vi "SMO.TopLevel.TestLauncher.vi"() -> ()   [LabVIEW 2013]
uses:
  src/SMO/Typedefs/SMOState --Enum.ctl
  SMO.TopLevel.lvclass
  src/SMO/SMO.lvclass
  src/Registry/Registry-SMO.lvclass
panel:
  in  "Registered SMOs":i32(listbox)
  in  "Check Context":bool
  out "A Name":string
  in  "Start Nested":bool
  in  "Stop":bool
  # "SMO Test Launcher"
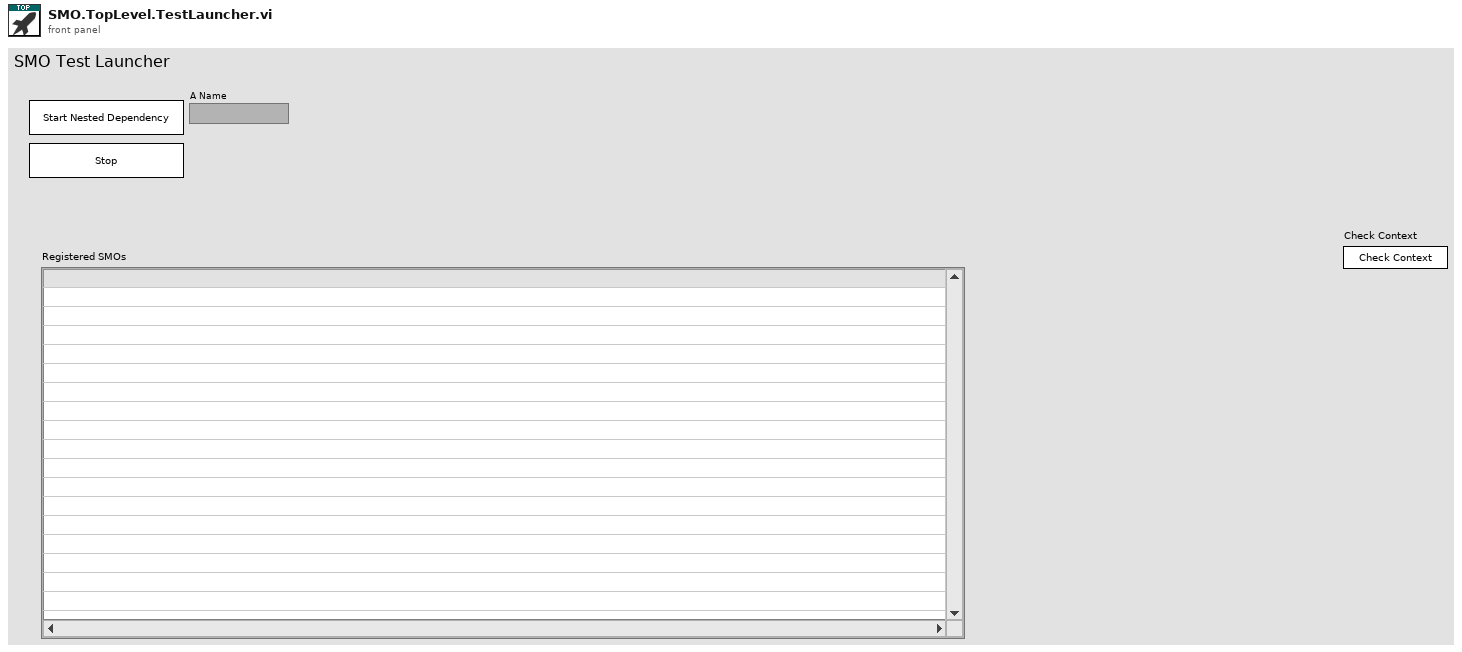
[diagram p1: front panel]
types:
  T1 = typedef "SMO.lvclass/SMOState --Enum.ctl" = enum16{"unknown", "Created", "Started", "Stopped"}
  T2 = enum32{"invalid app kind", "Development System", "Run Time System", "Student Edition", "Embedded LabVIEW", "Evaluation", "Custom"}
  T3 = enum32{"Invalid", "Standard", "Closed", "Hidden", "Minimized", "Maximized"}
  T4 = cluster{"Core":cluster{"Current VI Reference":refnum<vi>, "Close Panel on Exit?":bool}, "SMO":refnum<class "SMO.TopLevel.lvclass">, "Your string data":string}
  T5 = cluster{"Current VI Reference":refnum<vi>, "Close Panel on Exit?":bool}
  T6 = typedef "Registry-SMO.lvclass/PublicRegistryEvents--Cluster.ctl" = cluster{"Register Event":refnum<user-event>, "Unregister Event":refnum<user-event>}
  T7 = typedef "SMO.lvclass/Public Events.ctl" = cluster{"Error":refnum<user-event>, "State":refnum<user-event>}
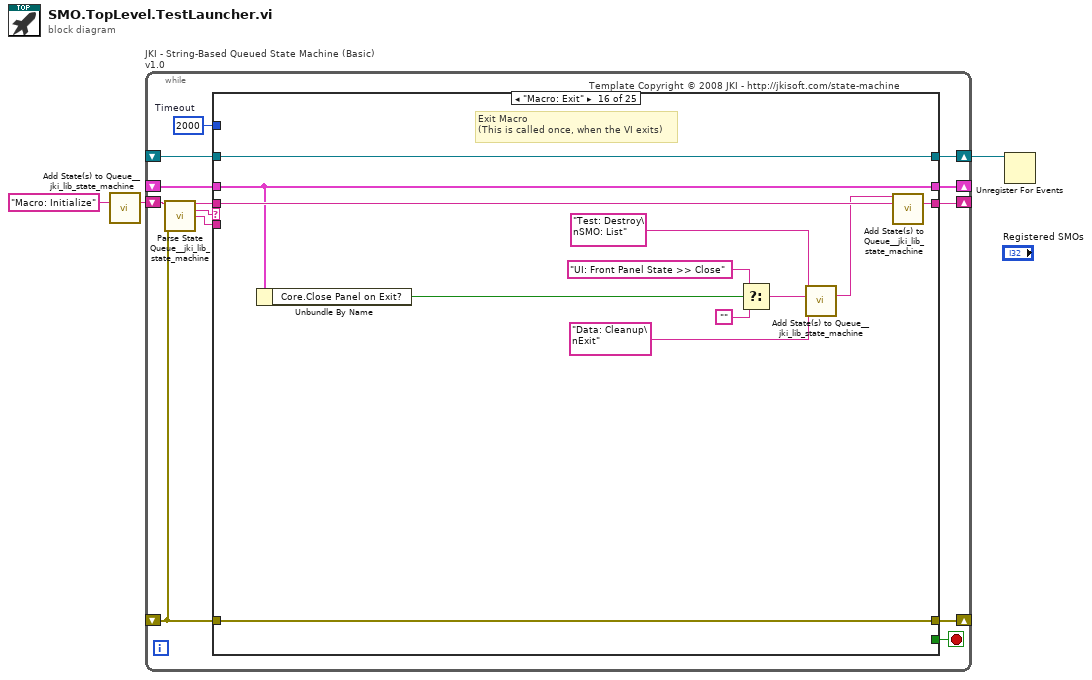
[diagram p0: block diagram]
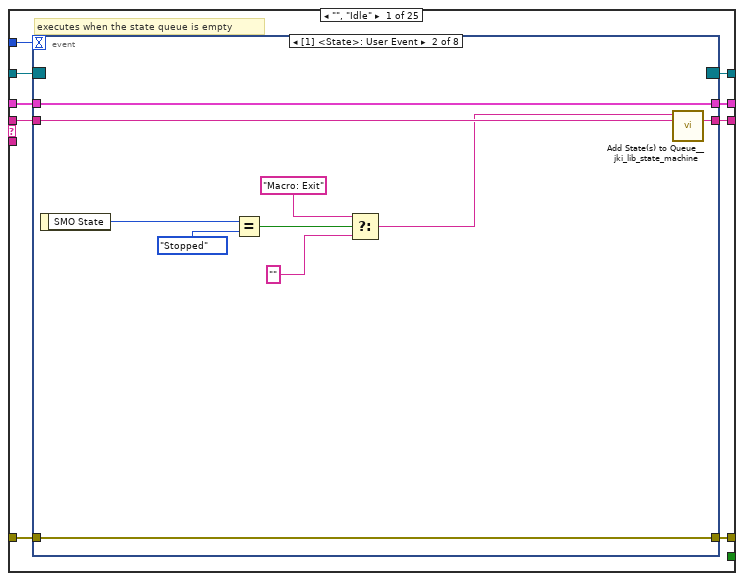
[diagram p2: hidden frame]
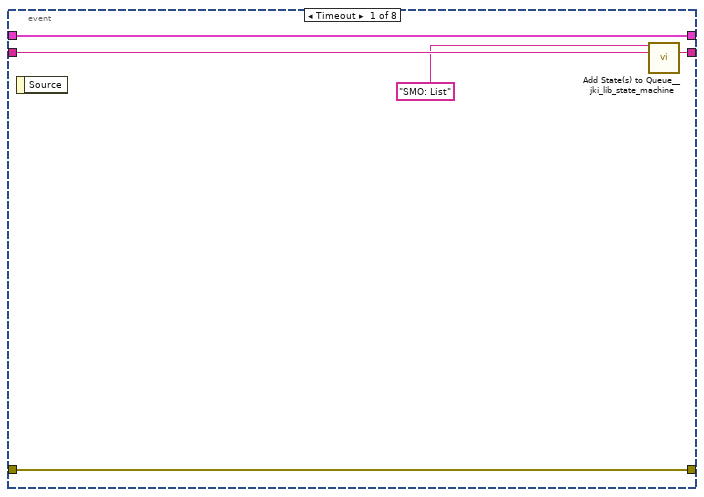
[diagram p3: hidden frame]
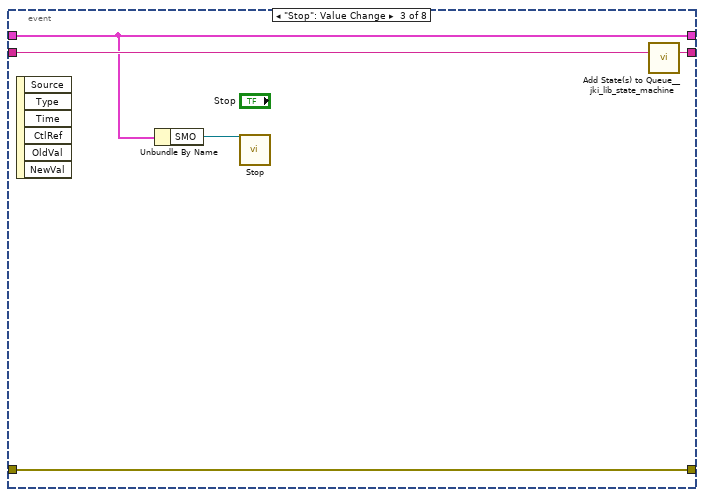
[diagram p4: hidden frame]
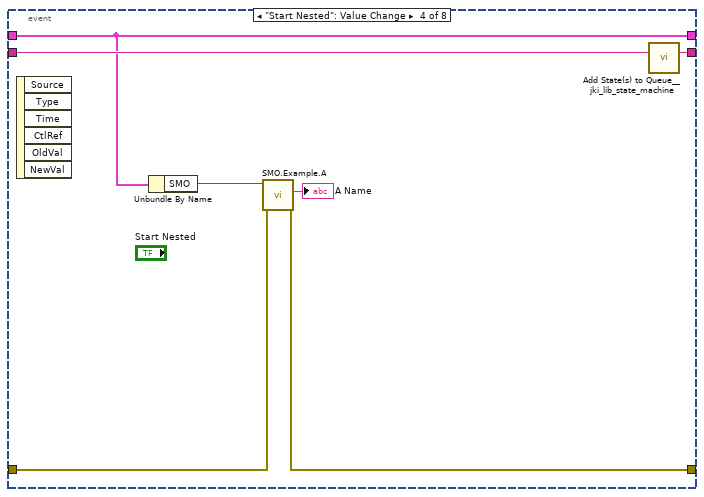
[diagram p5: hidden frame]
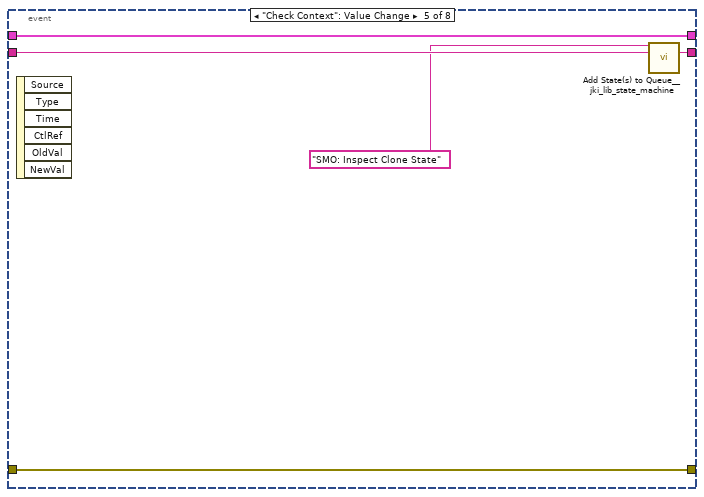
[diagram p6: hidden frame]
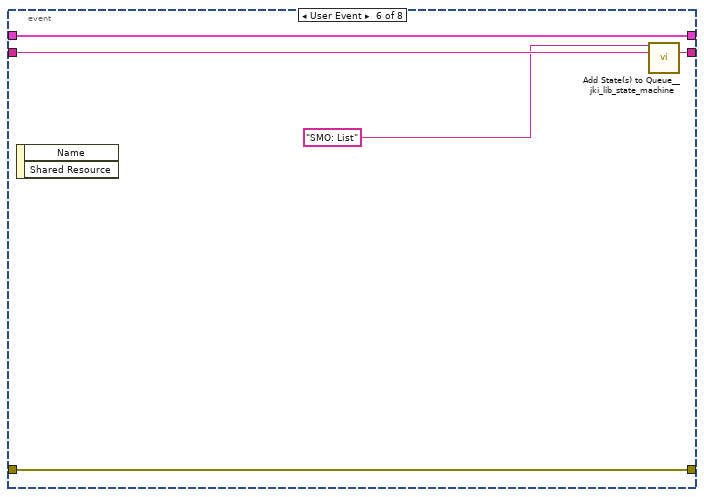
[diagram p7: hidden frame]
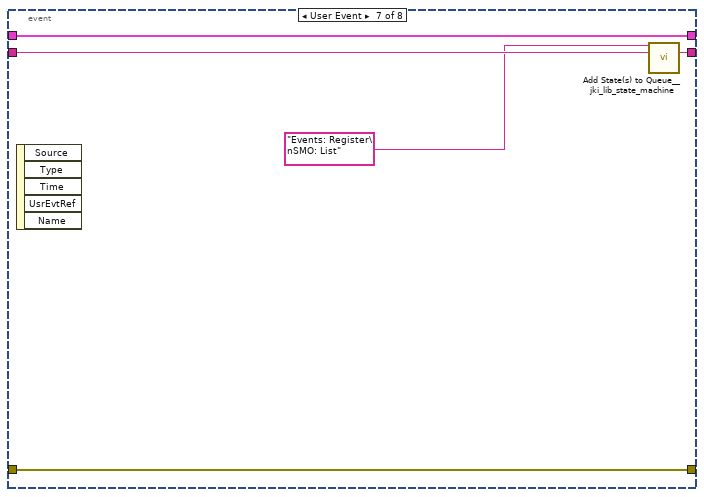
[diagram p8: hidden frame]
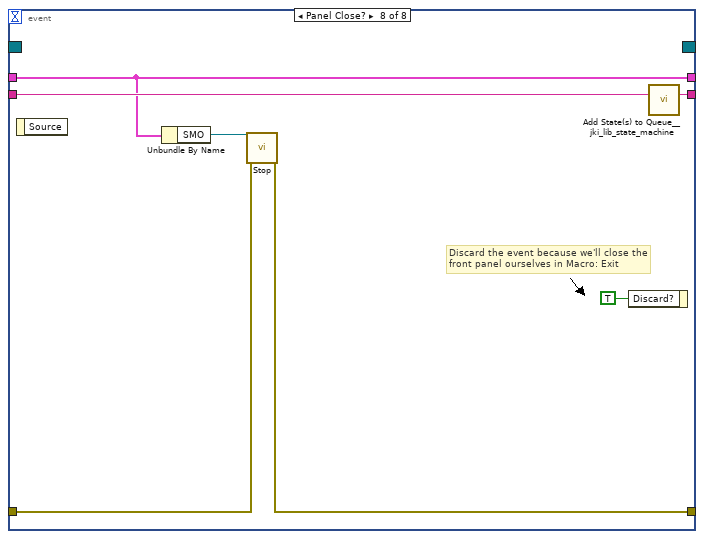
[diagram p9: hidden frame]
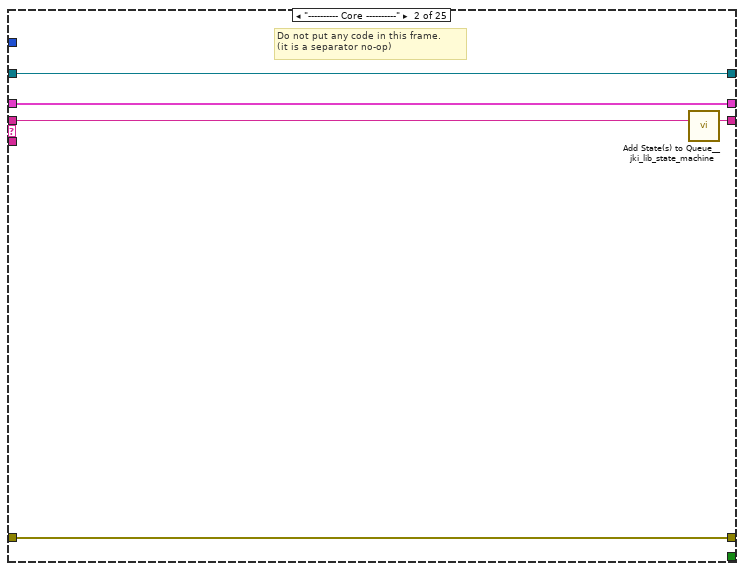
[diagram p10: hidden frame]
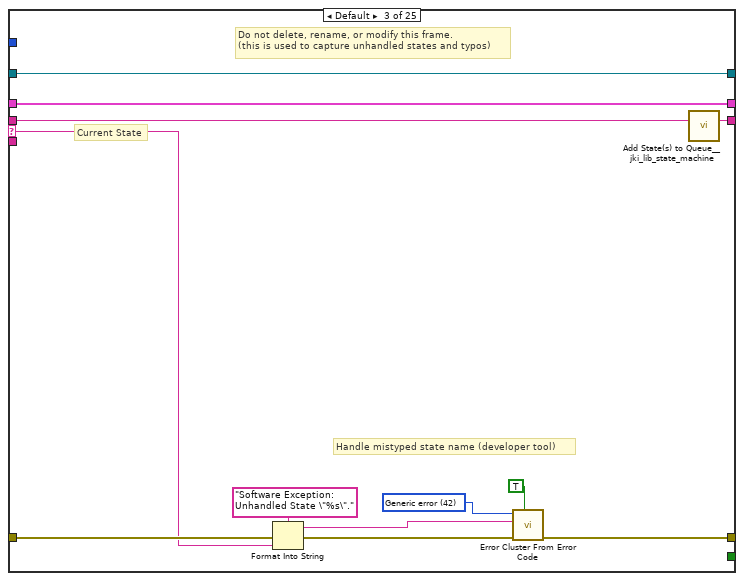
[diagram p11: hidden frame]
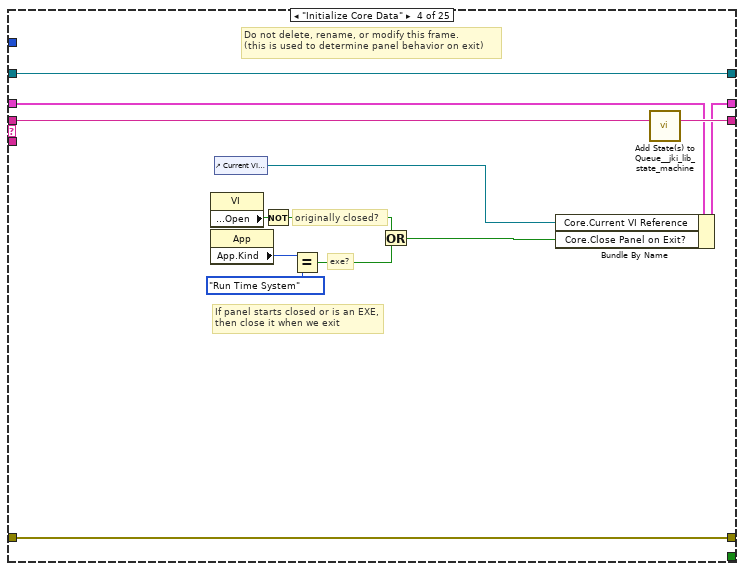
[diagram p12: hidden frame]
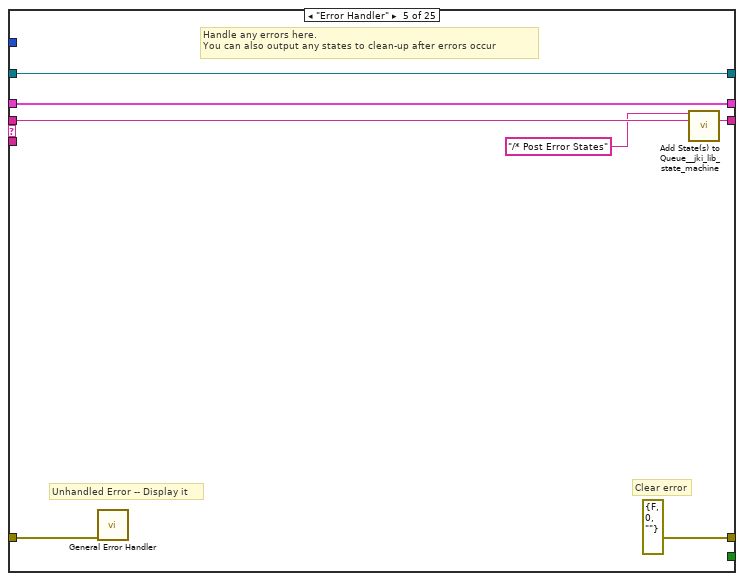
[diagram p13: hidden frame]
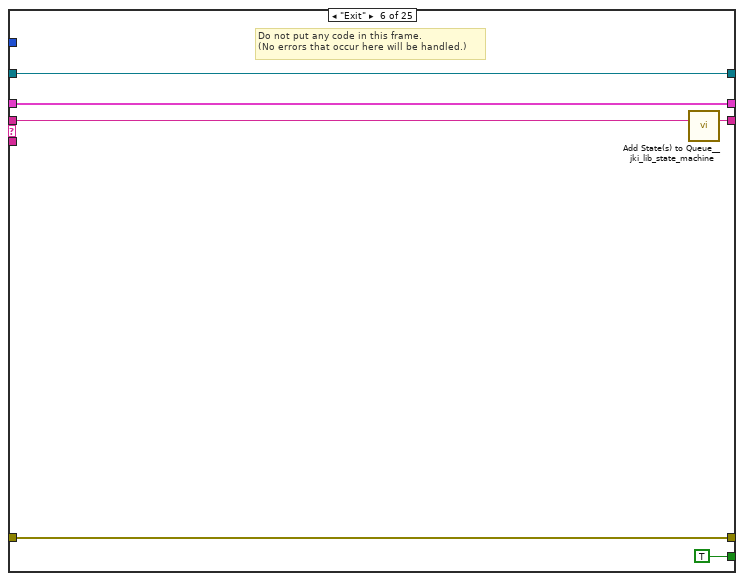
[diagram p14: hidden frame]
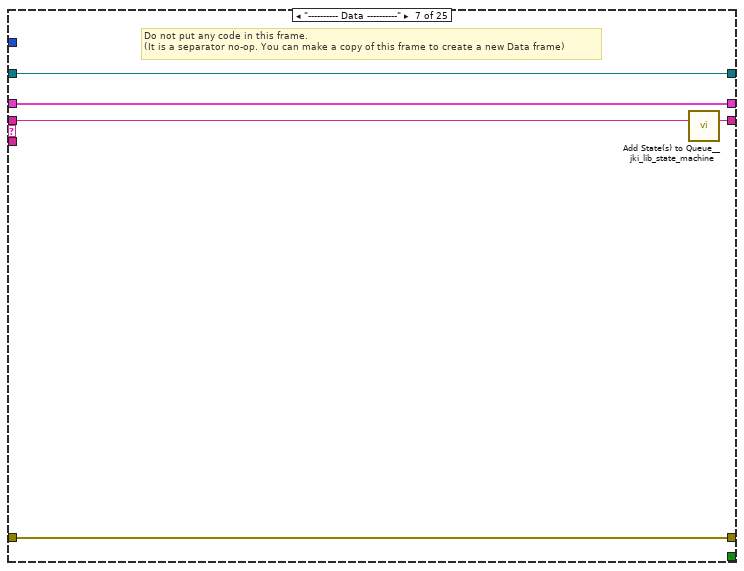
[diagram p15: hidden frame]
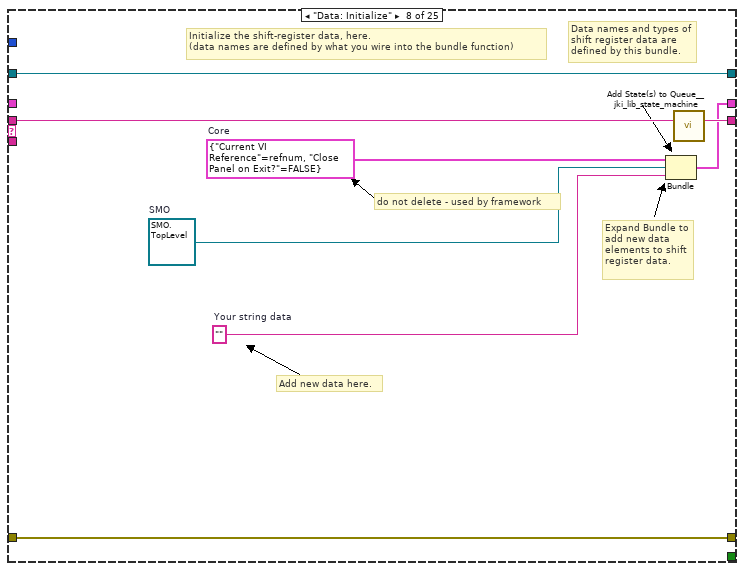
[diagram p16: hidden frame]
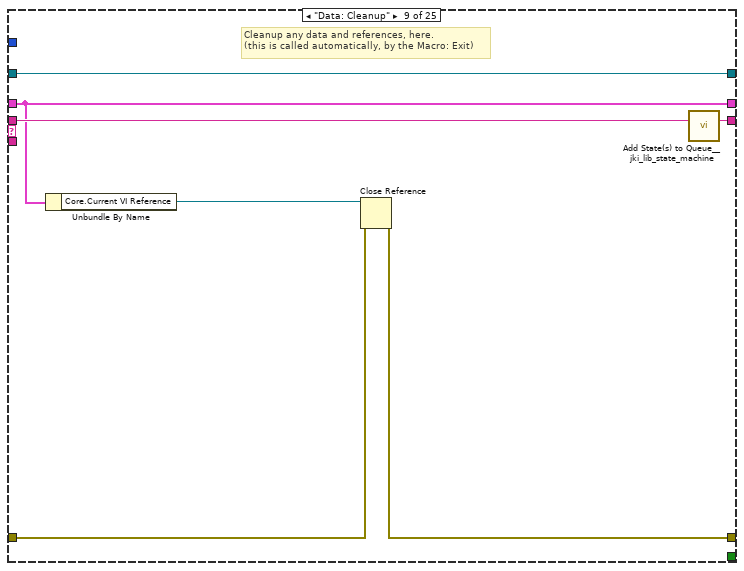
[diagram p17: hidden frame]
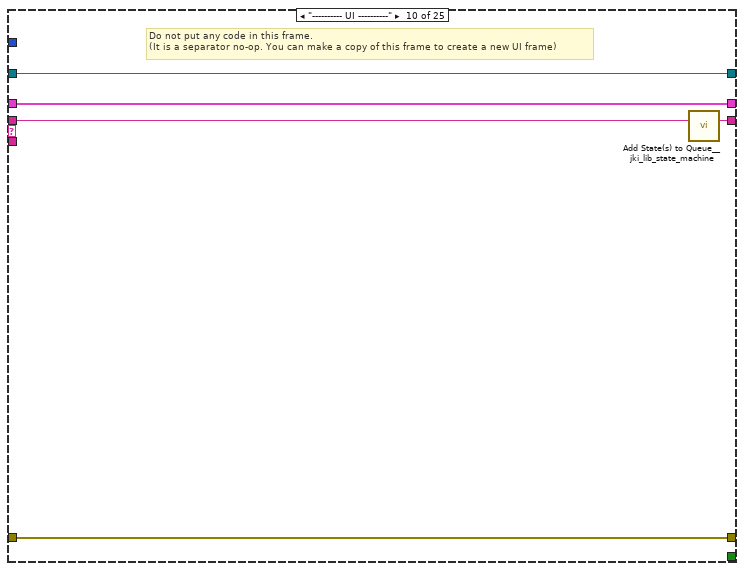
[diagram p18: hidden frame]
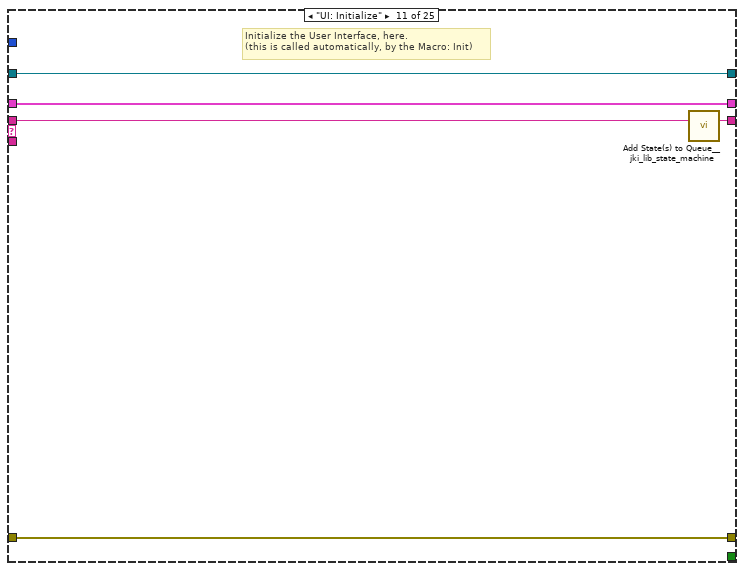
[diagram p19: hidden frame]
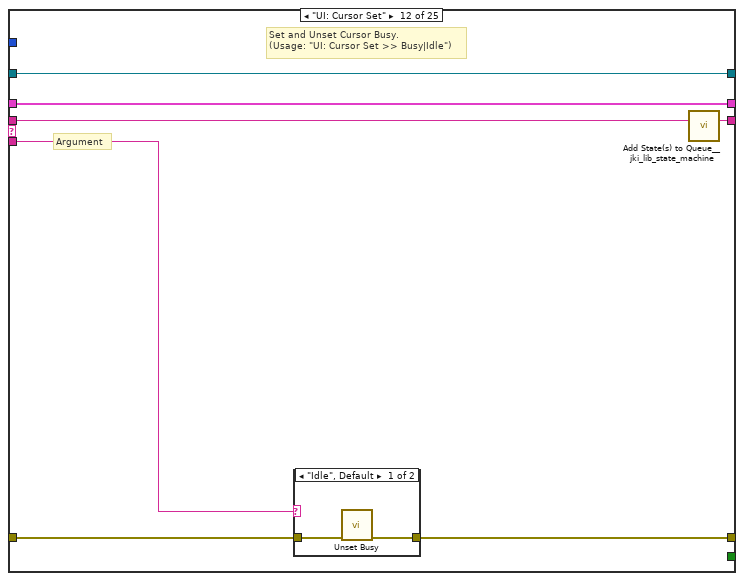
[diagram p20: hidden frame]
diagram:
  n1 = call <vilib>:"Add State(s) to Queue__jki_lib_state_machine.vi"("State(s) in (\"\")"="Macro: Initialize") -> ("States Out"=w1:string)  [unwired: 14 in]
  n2 = while "JKI - String-Based Queued State Machine (Basic) v1.0" {
    shift-right: [w9] -> _
    shift-left: _ -> [w8]
    shift-right: [w12] -> _
    shift-left: _ -> [w6]
    shift-right: [w11] -> _
    shift-left: w1 -> [w13]
    shift-right: [w4] -> w3
    shift-left: _ -> [w5]
    stop <- w10 stop-if-true
    w7 = 2000  # Timeout
    # "Template Copyright © 2008 JKI - http://jkisoft.com/state-machine"
    n3 = call <vilib>:"Parse State Queue__jki_lib_state_machine.vi"("State Queue"=w13, "Error In (no error)"=w6) -> ("Remaining States"=w15:string, "Current State"=w16:string, "Arguments"=w14:string)  [unwired: 11 in]
    n4 = case shown="\"Macro: Exit\"" w16 {
      selector: w16 -> [_ _ w81 _ _ _ _ _ _ _ _ _ _ _ _ _ _ _ _ _ _ _ _ _ _]
      tunnel: w15 -> [w25 w79 w85 w104 w111 w117 w122 w130 w137 w142 w147 w154 w166 w193 w199 w211 w216 w221 w226 w240 w249 w258 w263 w270 w293]
      tunnel: w14 -> [_ _ _ _ _ _ _ _ _ _ _ w149 w160 _ _ _ _ _ _ _ _ _ _ _ _]
      tunnel: w8 -> [w23 w76 w83 w95 w108 w115 w119 _ w132 w139 w145 w152 w162 w190 w196 w208 w213 w219 w223 w237 w245 w254 w260 w265 w290]
      tunnel: [w22 w77 w87 w101 errorcluster {"status"=FALSE, "code"=0, "source"=""} ("error out") w114 w120 w127 w133 w140 w144 w150 w163 w191 w197 w209 w214 w217 w224 w231 w241 w250 w261 w268 w291] -> w12
      tunnel: w6 -> [w21 w77 w86 w101 w107 w114 w120 w127 w134 w140 w144 w151 w164 w191 w197 w209 w214 w217 w224 w232 w242 w251 w261 w268 w291]
      tunnel: [w24 w78 w84 w103 w110 w116 w121 w129 w136 w141 w146 w153 w165 w192 w198 w210 w215 w220 w225 w239 w248 w257 w262 w269 w292] -> w11
      tunnel: [_ _ _ _ _ TRUE _ _ _ _ _ _ _ _ _ _ _ _ _ _ _ _ _ _ _] -> w10
      tunnel: [w20 w76 w83 w102 w108 w115 w119 w128 w132 w139 w145 w152 w162 w190 w196 w208 w213 w219 w223 w236 w247 w256 w260 w265 w290] -> w9
      tunnel: w7 -> [w19 _ _ _ _ _ _ _ _ _ _ _ _ _ _ _ _ _ _ _ _ _ _ _ _]
      tunnel: w5 -> [w18 w75 w80 w92 w105 w112 w118 w124 w131 w138 w143 w148 w159 w189 w194 w201 w212 w218 w222 _ w246 w255 w259 w264 w289]
      tunnel: [w17 w75 w80 w92 w105 w112 w118 w124 w131 w138 w143 w148 w159 w189 w194 w201 w212 w218 w222 w229 w246 w255 w259 w264 w289] -> w4
      frame "", "Idle" {
        # "executes when the state queue is empty"
        n5 = event shown="[1] <State>: User Event" {
          selector: w18 -> [_ _ _ _ _ _ _ _]
          dyn-events: [_ _ _ _ _ _ _ _] -> w17
          timeout: w19 -> [_ _ _ _ _ _ _ _]
          tunnel: w25 -> [w30 w40 w45 w52 w57 w62 w67 w74]
          tunnel: [w29 w39 w44 w51 w56 w61 w66 w73] -> w24
          tunnel: w23 -> [w27 w37 w42 w49 w54 w59 w64 w70]
          tunnel: [w28 w38 w43 w46 w55 w60 w65 w68] -> w22
          tunnel: w21 -> [w28 w38 w43 w47 w55 w60 w65 w69]
          tunnel: [w27 w37 w42 w49 w54 w59 w64 w70] -> w20
          event Timeout {
            n6 = event-data() -> ()  [unwired: 1 in, 1 out]
            n7 = call <vilib>:"Add State(s) to Queue__jki_lib_state_machine.vi"("State(s) in Front (\"\")"="SMO: List", "State(s) in (\"\")"=w30) -> ("States Out"=w29:string)  [unwired: 13 in]
          }
          event User Event {
            n8 = event-data() -> ("SMO State"=w36:T1)  [unwired: 1 in]
            n9 = Equal?(x=w36, y=SMOState_--Enum."Stopped") -> (x = y?=w34:bool)
            n10 = Select(t="Macro: Exit", s=w34, f="") -> (s? t:f=w31:string)
            n11 = call <vilib>:"Add State(s) to Queue__jki_lib_state_machine.vi"("State(s) in Front (\"\")"=w31, "State(s) in (\"\")"=w40) -> ("States Out"=w39:string)  [unwired: 13 in]
          }
          event "Stop": Value Change {
            n12 = event-data() -> ()  [unwired: 1 in, 6 out]
            n13 = Unbundle By Name(w42) -> ("SMO"=w41:refnum<class "SMO.TopLevel.lvclass">)
            n14 = call "Stop.vi"("SMO"=w41) -> ()  [unwired: 9 in, 2 out]
            n15 = call <vilib>:"Add State(s) to Queue__jki_lib_state_machine.vi"("State(s) in (\"\")"=w45) -> ("States Out"=w44:string)  [unwired: 14 in]
          }
          event "Start Nested": Value Change {
            n16 = event-data() -> ()  [unwired: 1 in, 6 out]
            n17 = Unbundle By Name(w49) -> ("SMO"=w48:refnum<class "SMO.TopLevel.lvclass">)
            n18 = call "SMO.Example.A.vi"("error in (no error)"=w47, "SMO.Example"=w48) -> ("error out"=w46:errorcluster, "Nested Dependency Name"=→"A Name":string)  [unwired: 7 in, 1 out]
            n19 = call <vilib>:"Add State(s) to Queue__jki_lib_state_machine.vi"("State(s) in (\"\")"=w52) -> ("States Out"=w51:string)  [unwired: 14 in]
          }
          event "Check Context": Value Change {
            n20 = event-data() -> ()  [unwired: 1 in, 6 out]
            n21 = call <vilib>:"Add State(s) to Queue__jki_lib_state_machine.vi"("State(s) in Front (\"\")"="SMO: Inspect Clone State", "State(s) in (\"\")"=w57) -> ("States Out"=w56:string)  [unwired: 13 in]
          }
          event User Event {
            n22 = event-data() -> ()  [unwired: 1 in, 2 out]
            n23 = call <vilib>:"Add State(s) to Queue__jki_lib_state_machine.vi"("State(s) in Front (\"\")"="SMO: List", "State(s) in (\"\")"=w62) -> ("States Out"=w61:string)  [unwired: 13 in]
          }
          event User Event {
            n24 = event-data() -> ()  [unwired: 1 in, 5 out]
            n25 = call <vilib>:"Add State(s) to Queue__jki_lib_state_machine.vi"("State(s) in Front (\"\")"="Events: Register\nSMO: List", "State(s) in (\"\")"=w67) -> ("States Out"=w66:string)  [unwired: 13 in]
          }
          event Panel Close? {
            # "Discard the event because we'll close the front panel ourselves in Macro: Exit"
            n26 = event-data() -> ()  [unwired: 1 in, 1 out]
            n27 = Unbundle By Name(w70) -> ("SMO"=w71:refnum<class "SMO.TopLevel.lvclass">)
            n28 = call "Stop.vi"("error in (no error)"=w69, "SMO"=w71) -> ("error out"=w68:errorcluster)  [unwired: 8 in, 1 out]
            n29 = event-data("Discard?"=TRUE) -> ()  [unwired: 1 in, 1 out]
            n30 = call <vilib>:"Add State(s) to Queue__jki_lib_state_machine.vi"("State(s) in (\"\")"=w74) -> ("States Out"=w73:string)  [unwired: 14 in]
          }
        }
      }
      frame "---------- Core ----------" {
        # "Do not put any code in this frame.\n(it is a separator no-op)"
        n31 = call <vilib>:"Add State(s) to Queue__jki_lib_state_machine.vi"("State(s) in (\"\")"=w79) -> ("States Out"=w78:string)  [unwired: 14 in]
      }
      frame Default {
        w90 = 42 items=["No error", "Argument error", "Memory is full", "Out of zone", "End of file", "File already open", "Generic file I/O error", "File not found", "File permission error", "Disk is full", "Duplicate path", "Too many files open", "System feature not enabled", "Resource file not found", "Cannot add resource", "Resource not found", "Image not found", "Image memory error", "Pen does not exist", "Config type invalid", "Config token not found", "Config parse error", "Config memory error", "Bad external code format", "Bad external code offset", "External code not present", "Null window", "Destroy window error", "Null menu", "Print aborted", "Bad print record", "Print driver error", "Windows error during printing", "Memory error during printing", "Print dialog error", "Generic print error", "Invalid device refnum", "Device not found", "Device parameter error", "Device unit error", "Cannot open device", "Device call aborted", "Generic error", "Cancelled by user", "Object ID too low", "Object ID too high", "Object not in heap", "Unknown heap", "Unknown object (invalid DefProc)", "Unknown object (DefProc not in table)", "Message out of range", "Invalid (null) method", "Unknown message", "Manager call not supported", "Bad address", "Network operation in progress", "Network operation timed out", "Connection is busy", "Network attribute not supported", "Network error", "Address in use", "System out of memory", "Connection aborted", "Connection refused", "Not connected", "Already connected", "Connection closed", "Initialization error (interapplication manager)", "Bad occurrence", "Wait on unbound occurrence handler", "Occurrence queue overflow", "Datalog type conflict", "Unused", "Unrecognized type (interapplication manager)", "Memory corrupt", "Failed to make temporary DLL", "Old CIN version", "Drag socket not found", "Failed to load drop-object", "Failed to register OLE object", "Failed to release OLE object", "Format specifier type mismatch", "Unknown format specifier", "Too few format specifiers", "Too many format specifiers", "Scan failed", "Newer CIN version", "Error converting to variant", "Runtime menu error", "Password tampered", "Variant attribute not found", "Incompatible variant data type", "Event data is not available", "Event Store is not present", "Occurrence is not found", "Event Queue is not created", "Event info is not available", "Refnum passed is NULL", "Error retrieving Class GUID", "Error retrieving CoClass GUID", "Error retrieving TypeLib GUID.", "Bad built application magic bytes.", "Specific driver is different from the specific driver associated with the Logical Name.", "There is no session opened to the class driver.", "Max Error", "MAX - Error with config objects", "MAX - Error loading configuration", "MAX - Group not supported"]
        # "Current State"
        # "Do not delete, rename, or modify this frame.\n(this is used to capture unhandled states and typos)"
        # "Handle mistyped state name (developer tool)"
        n32 = Format Into String(format string="Software Exception: Unhandled State \"%s\"." ("message"), error in=w86, w81) -> (resulting string=w89:string, error out=w88:errorcluster)  [unwired: 1 in]
        n33 = call <vilib>:"Error Cluster From Error Code.vi"("show call chain? (False)"=TRUE, "error in (no error)"=w88, "error message (\"\")"=w89, "error code (0)"=w90) -> ("error out"=w87:errorcluster)  [unwired: 5 in]
        n34 = call <vilib>:"Add State(s) to Queue__jki_lib_state_machine.vi"("State(s) in (\"\")"=w85) -> ("States Out"=w84:string)  [unwired: 14 in]
      }
      frame "Initialize Core Data" {
        # "Do not delete, rename, or modify this frame.\n(this is used to determine panel behavior on exit)"
        # "originally closed?"
        # "exe?"
        # "If panel starts closed or is an EXE, then close it when we exit"
        n35 = property class="VI"() -> ("Front Panel.Open"=w100:bool)  [unwired: 2 in, 2 out]
        n36 = property class="App"() -> ("App.Kind"=w99:T2)  [unwired: 2 in, 2 out]
        n37 = control-ref of="Current VI Reference"() -> (w93:refnum<vi>)
        n38 = Not(x=w100) -> (.not. x?=w97:bool)
        n39 = Equal?(x=w99, y=T2."Run Time System" ("Application:Kind")) -> (x = y?=w96:bool)
        n40 = Or(x=w97, y=w96) -> (x .or. y?=w94:bool)
        n41 = Bundle By Name(cluster=w95, "Core.Current VI Reference"=w93, "Core.Close Panel on Exit?"=w94) -> (w102:T4)
        n42 = call <vilib>:"Add State(s) to Queue__jki_lib_state_machine.vi"("State(s) in (\"\")"=w104) -> ("States Out"=w103:string)  [unwired: 14 in]
      }
      frame "Error Handler" {
        # "Unhandled Error -- Display it"
        # "Handle any errors here.\nYou can also output any states to clean-up after errors occur"
        # "Clear error"
        n43 = call <vilib>:"General Error Handler.vi"("error in (no error)"=w107) -> ()  [unwired: 10 in, 5 out]
        n44 = call <vilib>:"Add State(s) to Queue__jki_lib_state_machine.vi"("State(s) in Front (\"\")"="/* Post Error States", "State(s) in (\"\")"=w111) -> ("States Out"=w110:string)  [unwired: 13 in]
      }
      frame "Exit" {
        # "Do not put any code in this frame.\n(No errors that occur here will be handled.)"
        n45 = call <vilib>:"Add State(s) to Queue__jki_lib_state_machine.vi"("State(s) in (\"\")"=w117) -> ("States Out"=w116:string)  [unwired: 14 in]
      }
      frame "---------- Data ----------" {
        # "Do not put any code in this frame.\n(It is a separator no-op. You can make a copy of this frame to create a new Data frame)"
        n46 = call <vilib>:"Add State(s) to Queue__jki_lib_state_machine.vi"("State(s) in (\"\")"=w122) -> ("States Out"=w121:string)  [unwired: 14 in]
      }
      frame "Data: Initialize" {
        w123 = refnum<class "SMO.TopLevel.lvclass"> refnum  # SMO
        w125 = T5 {"Current VI Reference"=refnum, "Close Panel on Exit?"=FALSE}  # Core
        w126 = ""  # Your string data
        # "do not delete - used by framework"
        # "Expand Bundle to add new data elements to shift register data."
        # "Add new data here."
        # "Data names and types of shift register data are defined by this bundle."
        # "Initialize the shift-register data, here.\n(data names are defined by what you wire into the bundle function)"
        n47 = Bundle("Core"=w125, "SMO"=w123, "Your string data"=w126) -> (w128:T4)  [unwired: 1 in]
        n48 = call <vilib>:"Add State(s) to Queue__jki_lib_state_machine.vi"("State(s) in (\"\")"=w130) -> ("States Out"=w129:string)  [unwired: 14 in]
      }
      frame "Data: Cleanup" {
        # "Cleanup any data and references, here.\n(this is called automatically, by the Macro: Exit)"
        n49 = Unbundle By Name(w132) -> ("Core.Current VI Reference"=w135:refnum<vi>)
        n50 = Close Reference(reference=w135, error in (no error)=w134) -> (error out=w133:errorcluster)
        n51 = call <vilib>:"Add State(s) to Queue__jki_lib_state_machine.vi"("State(s) in (\"\")"=w137) -> ("States Out"=w136:string)  [unwired: 14 in]
      }
      frame "---------- UI ----------" {
        # "Do not put any code in this frame.\n(It is a separator no-op. You can make a copy of this frame to create a new UI frame)"
        n52 = call <vilib>:"Add State(s) to Queue__jki_lib_state_machine.vi"("State(s) in (\"\")"=w142) -> ("States Out"=w141:string)  [unwired: 14 in]
      }
      frame "UI: Initialize" {
        # "Initialize the User Interface, here.\n(this is called automatically, by the Macro: Init)"
        n53 = call <vilib>:"Add State(s) to Queue__jki_lib_state_machine.vi"("State(s) in (\"\")"=w147) -> ("States Out"=w146:string)  [unwired: 14 in]
      }
      frame "UI: Cursor Set" {
        # "Argument"
        # "Set and Unset Cursor Busy.\n(Usage: \"UI: Cursor Set >> Busy|Idle\")"
        n54 = case shown="\"Idle\", Default" w149 {
          tunnel: w151 -> [w156 w158]
          tunnel: [w155 w157] -> w150
          frame "Idle", Default {
            n55 = call <vilib>:"Unset Busy.vi"("error in (no error)"=w156) -> ("error out"=w155:errorcluster)  [unwired: 10 in]
          }
          frame "Busy" {
            n56 = call <vilib>:"Set Busy.vi"("error in (no error)"=w158) -> ("error out"=w157:errorcluster)  [unwired: 9 in, 1 out]
          }
        }
        n57 = call <vilib>:"Add State(s) to Queue__jki_lib_state_machine.vi"("State(s) in (\"\")"=w154) -> ("States Out"=w153:string)  [unwired: 14 in]
      }
      frame "UI: Front Panel State" {
        # "Argument"
        # "Set Front Panel Open or Closed\n(Usage: \"UI: Front Panel State >> Open|Close\")"
        n58 = Unbundle By Name(w162) -> ("Core.Current VI Reference"=w161:refnum<vi>)
        n59 = case shown="\"Open\", Default" w160 {
          tunnel: w164 -> [w170 w183]
          tunnel: [w172 w184] -> w163
          tunnel: w161 -> [w171 w181]
          frame "Open", Default {
            n60 = property class="VI"(reference=w171, error in=w170) -> (reference out=w168:refnum<vi>, error out=w169:errorcluster, "Front Panel.Open"=w167:bool)
            n61 = case shown="False" w167 {
              tunnel: [w175 w178] -> w172
              tunnel: w169 -> [w174 w178]
              tunnel: w168 -> [w173 _]
              frame False {
                n62 = invoke class="VI" method="FP.Open"(reference=w173, error in=w174, "Activate"=TRUE, "State"=T3."Standard") -> (error out=w175:errorcluster)  [unwired: 1 in, 4 out]
              }
              frame True {
              }
            }
          }
          frame "Close" {
            n63 = property class="VI"(reference=w181, error in=w183) -> (reference out=w180:refnum<vi>, error out=w182:errorcluster, "Front Panel.Open"=w179:bool)
            n64 = case shown="True" w179 {
              tunnel: [w185 w188] -> w184
              tunnel: w182 -> [w185 w187]
              tunnel: w180 -> [_ w186]
              frame False {
              }
              frame True {
                n65 = invoke class="VI" method="FP.Close"(reference=w186, error in=w187) -> (error out=w188:errorcluster)  [unwired: 1 in, 2 out]
              }
            }
          }
        }
        n66 = call <vilib>:"Add State(s) to Queue__jki_lib_state_machine.vi"("State(s) in (\"\")"=w166) -> ("States Out"=w165:string)  [unwired: 14 in]
      }
      frame "---------- Macro ----------" {
        # "Do not put any code in this frame.\n(It is a separator no-op. You can make a copy of this frame to create a new Macro frame)"
        n67 = call <vilib>:"Add State(s) to Queue__jki_lib_state_machine.vi"("State(s) in (\"\")"=w193) -> ("States Out"=w192:string)  [unwired: 14 in]
      }
      frame "Macro: Initialize" {
        w195 = "Data: Initialize\nInitialize Core Data\nUI: Initialize\nUI: Front Panel State >> Open\n\nTest: Create\nSMO: List\nTest: Start"  # Data: Initialize Initialize Core Data UI: Initialize UI: Front Panel State >> Open  Test: Create SMO: List Test: Start
        # "Initialization Macro\n(This is called once, when the VI starts)"
        n68 = call <vilib>:"Add State(s) to Queue__jki_lib_state_machine.vi"("State(s) in Front (\"\")"=w195, "State(s) in (\"\")"=w199) -> ("States Out"=w198:string)  [unwired: 13 in]
      }
      frame "Macro: Exit" {
        # "Exit Macro\n(This is called once, when the VI exits)"
        n69 = Unbundle By Name(w208) -> ("Core.Close Panel on Exit?"=w207:bool)
        n70 = Select(t="UI: Front Panel State >> Close", s=w207, f="") -> (s? t:f=w204:string)
        n71 = call <vilib>:"Add State(s) to Queue__jki_lib_state_machine.vi"("State(s) in Front (\"\")"="Test: Destroy\nSMO: List", "State(s) in (\"\")"=w204, "State(s) at Back (\"\")"="Data: Cleanup\nExit") -> ("States Out"=w202:string)  [unwired: 12 in]
        n72 = call <vilib>:"Add State(s) to Queue__jki_lib_state_machine.vi"("State(s) in Front (\"\")"=w202, "State(s) in (\"\")"=w211) -> ("States Out"=w210:string)  [unwired: 13 in]
      }
      frame "---------- Events ----------" {
        n73 = call <vilib>:"Add State(s) to Queue__jki_lib_state_machine.vi"("State(s) in (\"\")"=w216) -> ("States Out"=w215:string)  [unwired: 14 in]
      }
      frame "Events: Register" {
        n74 = call <vilib>:"Add State(s) to Queue__jki_lib_state_machine.vi"("State(s) in (\"\")"=w221) -> ("States Out"=w220:string)  [unwired: 14 in]
      }
      frame "---------- Test ----------" {
        n75 = call <vilib>:"Add State(s) to Queue__jki_lib_state_machine.vi"("State(s) in (\"\")"=w226) -> ("States Out"=w225:string)  [unwired: 14 in]
      }
      frame "Test: Create" {
        n76 = call "Get Public Registry Events.vi"() -> ("Public Registry Events"=w227:T6)  [unwired: 10 in, 1 out]
        n77 = call "Create.vi"("error in (no error)"=w232, "SMO"=refnum<class "SMO.TopLevel.lvclass"> refnum ("SMO.Example.lvclass")) -> ("error out"=w233:errorcluster, "SMO out"=w235:refnum<class "SMO.TopLevel.lvclass">)  [unwired: 7 in, 1 out]
        n78 = call "GetPublicEvents.vi"("error in (no error)"=w233, "SMO"=w235) -> ("error out"=w231:errorcluster, "Public Events"=w230:T7, "SMO out"=w234:refnum<class "SMO.TopLevel.lvclass">)  [unwired: 7 in]
        n79 = Unbundle By Name(w230) -> ("State"=w228:refnum<user-event>)
        n80 = register-events(w227, w228) -> (reference out=w229:refnum<event-registration>)  [unwired: 2 in, 1 out]
        n81 = Bundle By Name(cluster=w237, "SMO"=w234) -> (w236:T4)
        n82 = call <vilib>:"Add State(s) to Queue__jki_lib_state_machine.vi"("State(s) in (\"\")"=w240) -> ("States Out"=w239:string)  [unwired: 14 in]
      }
      frame "Test: Start" {
        n83 = Unbundle By Name(w245) -> ("SMO"=w244:refnum<class "SMO.TopLevel.lvclass">)
        n84 = call "Start.vi"("error in (no error)"=w242, "SMO"=w244) -> ("error out"=w241:errorcluster, "SMO out"=w243:refnum<class "SMO.TopLevel.lvclass">)  [unwired: 8 in]
        n85 = Bundle By Name(cluster=w245, "SMO"=w243) -> (w247:T4)
        n86 = call <vilib>:"Add State(s) to Queue__jki_lib_state_machine.vi"("State(s) in (\"\")"=w249) -> ("States Out"=w248:string)  [unwired: 14 in]
      }
      frame "Test: Destroy" {
        n87 = Unbundle By Name(w254) -> ("SMO"=w253:refnum<class "SMO.TopLevel.lvclass">)
        n88 = call "Destroy.vi"("error in (no error)"=w251, "SMO"=w253) -> ("error out"=w250:errorcluster)  [unwired: 9 in]
        n89 = Bundle By Name(cluster=w254, "SMO"=refnum<class "SMO.TopLevel.lvclass"> refnum) -> (w256:T4)
        n90 = call <vilib>:"Add State(s) to Queue__jki_lib_state_machine.vi"("State(s) in (\"\")"=w258) -> ("States Out"=w257:string)  [unwired: 14 in]
      }
      frame "---------- SMO Registry ----------" {
        n91 = call <vilib>:"Add State(s) to Queue__jki_lib_state_machine.vi"("State(s) in (\"\")"=w263) -> ("States Out"=w262:string)  [unwired: 14 in]
      }
      frame "SMO: List" {
        n92 = call "List Subsystems.vi"() -> ("Subsystems"=w266:refnum<class "SMO.lvclass">[])  [unwired: 10 in, 1 out]
        n93 = for {
          tunnel: w266 -> [w275] mode=indexing
          tunnel: [w280] -> w267 mode=indexing
          tunnel: [w276] -> _ mode=indexing
          tunnel: [w272] -> _ mode=indexing
          tunnel: [w271] -> _ mode=indexing
          n94 = call "GetPublicEvents.vi"("SMO"=w275) -> ("Public Events"=w273:T7, "SMO out"=w274:refnum<class "SMO.lvclass">)  [unwired: 8 in, 1 out]
          n95 = Unbundle By Name(w273) -> ("Error"=w272:refnum<user-event>, "State"=w271:refnum<user-event>)
          n96 = call "Get Name.vi"("SMO"=w274) -> ("error out"=w279:errorcluster, "Name"=w284:string, "SMO out"=w288:refnum<class "SMO.lvclass">)  [unwired: 8 in]
          n97 = call "Get State.vi"("error in (no error)"=w279, "SMO"=w288) -> ("error out"=w278:errorcluster, "SMO State"=w285:T1, "SMO out"=w287:refnum<class "SMO.lvclass">)  [unwired: 7 in]
          n98 = Format Into String(w285) -> (resulting string=w283:string)  [unwired: 3 in, 1 out]
          n99 = call "Get GUID.vi"("error in (no error)"=w278, "SMO"=w287) -> ("error out"=w277:errorcluster, "GUID"=w281:string, "SMO out"=w286:refnum<class "SMO.lvclass">)  [unwired: 7 in]
          n100 = call "Get Qualified Name.vi"("error in (no error)"=w277, "SMO"=w286) -> ("error out"=w276:errorcluster, "Qualified Name"=w282:string)  [unwired: 7 in, 1 out]
          n101 = Build Array(w284, w283, w282, w281) -> (w280:string[])
        }
        n102 = property on="Registered SMOs" class="MCListbox (strict)"("ItemNames"=w267) -> ()  [unwired: 2 in, 2 out]
        n103 = call <vilib>:"Add State(s) to Queue__jki_lib_state_machine.vi"("State(s) in (\"\")"=w270) -> ("States Out"=w269:string)  [unwired: 14 in]
      }
      frame "SMO: Inspect Clone State" {
        n104 = property class="App" props=["App.AllVIs"]() -> ()  [unwired: 2 in, 3 out]
        n105 = call <vilib>:"Add State(s) to Queue__jki_lib_state_machine.vi"("State(s) in (\"\")"=w293) -> ("States Out"=w292:string)  [unwired: 14 in]
      }
    }
  }
  n106 = Unregister For Events(event registration refnum=w3) -> ()  [unwired: 1 in, 1 out]
